vi "Write pstrstates out.vi"(8 "error in (no error)":errorcluster, 10 "pstrstates out":T1, 11 "ZanClass in":refnum<class "ZanClass.lvclass">) -> (0 "error out":errorcluster, 3 "ZanClass out":refnum<class "ZanClass.lvclass">)   [LabVIEW 2019, in "ZanClass.lvclass"]
uses:
  ZanClass.lvclass
  ZanClass.lvclass/ZanClass.ctl
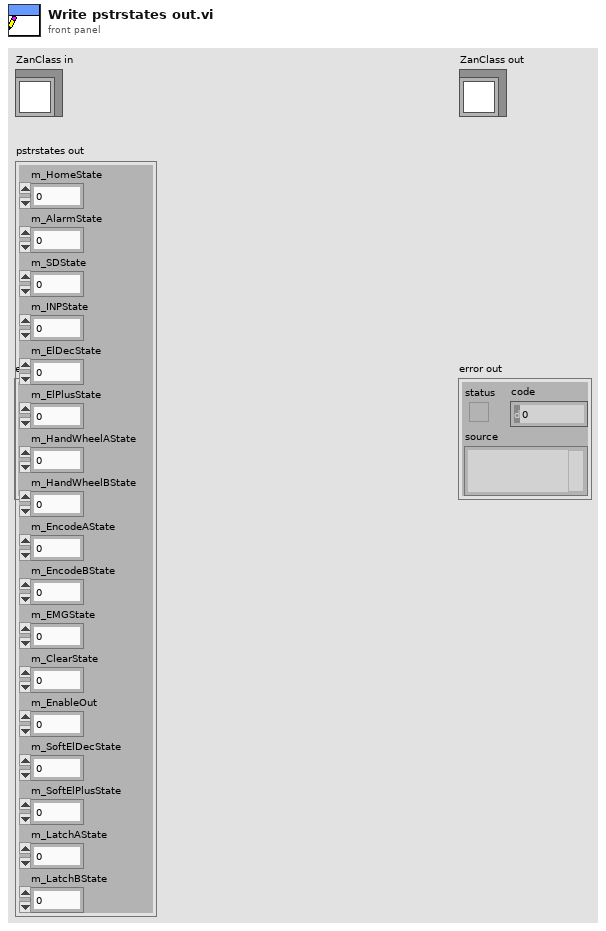
[diagram p1: front panel]
types:
  T1 = cluster{"m_HomeState":u8, "m_AlarmState":u8, "m_SDState":u8, "m_INPState":u8, "m_ElDecState":u8, "m_ElPlusState":u8, "m_HandWheelAState":u8, "m_HandWheelBState":u8, "m_EncodeAState":u8, "m_EncodeBState":u8, "m_EMGState":u8, "m_ClearState":u8, "m_EnableOut":u8, "m_SoftElDecState":u8, "m_SoftElPlusState":u8, "m_LatchAState":u8, "m_LatchBState":u8}
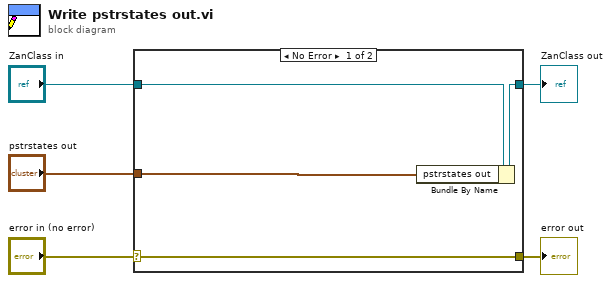
[diagram p0: block diagram]
diagram:
  n1 = case shown="No Error" "error in (no error)" {
    selector: "error in (no error)" -> [w9 w10]
    tunnel: [w9 w10] -> w4
    tunnel: [w7 w11] -> w2
    tunnel: "ZanClass in" -> [w8 w11]
    tunnel: "pstrstates out" -> [w6 _]
    frame No Error {
      n2 = Bundle By Name(cluster=w8, "pstrstates out"=w6) -> (w7:refnum<class "ZanClass.lvclass">)
    }
    frame Error {
    }
  }
  "error out" <- w4
  "ZanClass out" <- w2
